vi "Analyze Fan Speed (FPGA).vi"(10 "max fan speed threshold (RPM)":sgl, 11 "tacho RPM":sgl) -> (3 "max fan speed exceeded?":bool)   [LabVIEW 2014]
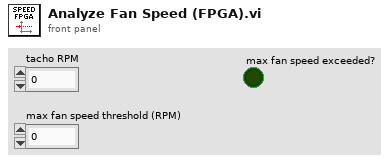
[diagram p1: front panel]
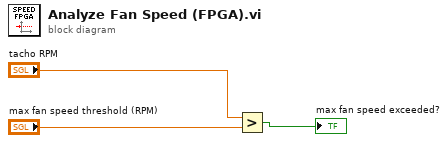
[diagram p0: block diagram]
diagram:
  n1 = Greater?(x="tacho RPM", y="max fan speed threshold (RPM)") -> (0:→"max fan speed exceeded?":bool)
